vi "UART Get Bytes Available.vi"(8 "Error In":errorcluster, 10 "UART Channel":u8, 11 "LINX Device Config":T1) -> (0 "Error Out":errorcluster, 1 "Bytes Availabe":u8, 3 "LINX Device Config":T1)   [LabVIEW 2011, in "LVH-LINX.lvlib" / "Device.lvlib"]
doc: "Get the number of bytes available in the specified UART channel receive buffer."
uses:
  Device.lvlib
  Type Defs/LINX Device Config.ctl
  Type Defs/Interface.ctl
  Type Defs/TCP Config.ctl
  Type Defs/Channels.ctl
  Type Defs/Error Type.ctl
  LVH-LINX.lvlib
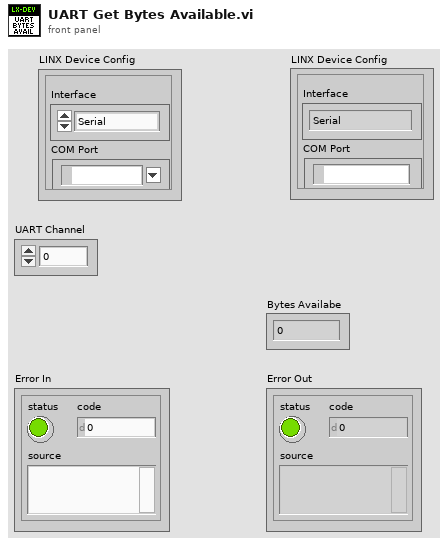
[diagram p1: front panel]
types:
  T1 = typedef "LVH-LINX.lvlib/Device.lvlib/LINX Device Config.ctl" = cluster{"Interface":T2, "COM Port":refnum<visa-resource-name>, "TCP Configuration":T3, "Device Family":u8, "Device ID":u8, "Device Name":string, "TCP Ref":refnum<k5>, "Channels":T4}
  T2 = typedef "LVH-LINX.lvlib/Interface.ctl" = enum16{"Serial", "TCP"}
  T3 = typedef "LVH-LINX.lvlib/Device.lvlib/TCP Config.ctl" = cluster{"IP Address":string, "Port":u16}
  T4 = typedef "LVH-LINX.lvlib/Channels.ctl" = cluster{"DI":u8[], "DO":u8[], "AI":u8[], "AO":u8[], "PWM":u8[], "QE":u8[], "UART":u8[], "I2C 2":u8[], "SPI":u8[], "CAN":u8[], "Servo":u8[], "AI Ref (V)":dbl, "AO Ref (V)":dbl, "AO Resolution (Bits)":u8}
  T5 = typedef "LVH-LINX.lvlib/Error Type.ctl" = enum16{"Unknown", "Timeout", "Corrupt Return Packet", "Unable To Connect", "Command Not Supported", "Channel DNE", "Invalid COM Config", "Firmware Version Mismatch", "myRIO Support", "CMD Specific Error"}
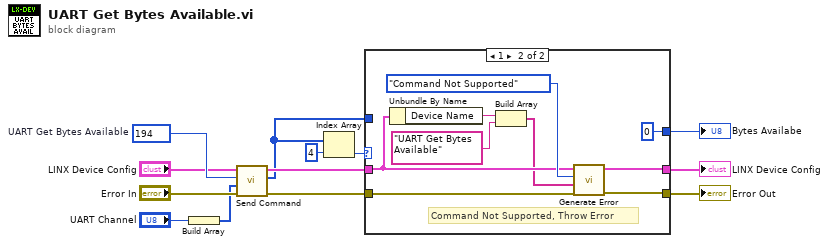
[diagram p0: block diagram]
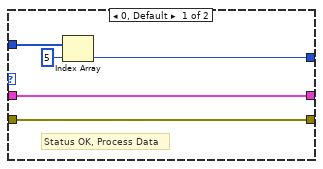
[diagram p2: hidden frame]
diagram:
  w12 = u16 194  # UART Get Bytes Available
  n1 = Build Array("UART Channel") -> (w3:u8[])
  n2 = call "Send Command.vi"("Error In"="Error In", "ARGS"=w3, "CMD"=w12, "LINX Device Config"="LINX Device Config") -> ("Error Out"=w5:errorcluster, "Response"=w2:u8[], "LINX Device Config"=w7:T1)  [unwired: 4 in, 1 out]
  n3 = Index Array(array=w2, index=4) -> (element=w9:u8)
  n4 = case shown="1" w9 {
    tunnel: [w18 w25] -> w8
    tunnel: w7 -> [w18 w21]
    tunnel: [w17 w26] -> w6
    tunnel: w5 -> [w17 w27]
    tunnel: w2 -> [w16 _]
    tunnel: [w14 u8 0 ("element")] -> w1
    frame 0, Default {
      # "Status OK, Process Data"
      n5 = Index Array(array=w16, index=5) -> (element=w14:u8)
    }
    frame 1 {
      # "Command Not Supported, Throw Error"
      n6 = Unbundle By Name(w21) -> ("Device Name"=w23:string)
      n7 = Build Array(w23, "UART Get Bytes Available") -> (w20:string[])
      n8 = call "Generate Error.vi"("Error In"=w27, "Arguments"=w20, "Error Type"=Error_Type."Command Not Supported", "LINX Device Config"=w21) -> ("Error Out"=w26:errorcluster, "LINX Device Config"=w25:T1)  [unwired: 6 in]
    }
  }
  "Error Out" <- w6
  "LINX Device Config" <- w8
  "Bytes Availabe" <- w1
